vi "Day 19-1.vi"() -> ()   [LabVIEW 2020]
uses:
  Vec3.ctl
panel:
  out "Sensors - 1":i32
  out "Iterations":i32
  out "Max Manhattan Distance":dbl
  out "Beacon Count":i32
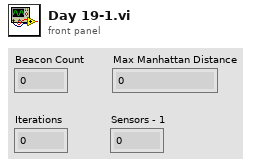
[diagram p1: front panel]
types:
  T1 = typedef "Vec3.ctl" = cluster{"X":dbl, "Y":dbl, "Z":dbl}
  T2 = typedef "Scanner.ctl" = cluster{"Position":T1, "Beacons":T1[]}
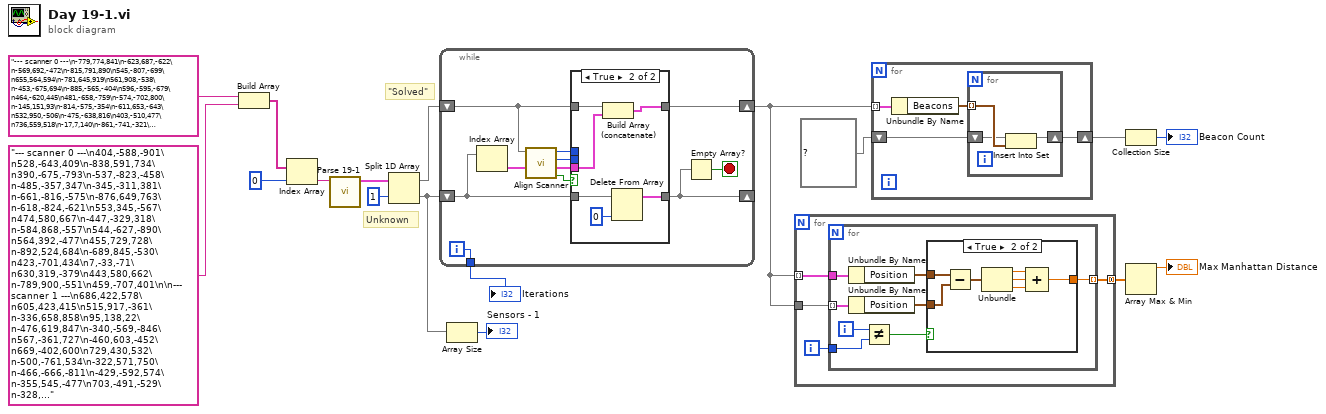
[diagram p0: block diagram]
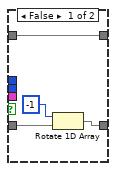
[diagram p3: hidden frame]
diagram:
  # "Unknown"
  # "\"Solved\""
  n1 = Build Array("--- scanner 0 ---\n-779,774,841\n-623,687,-622\n-569,692,-472\n-815,791,890\n545,-807,-699\n655,564,594\n-781,645,919\n561,908,-538\n-453,-675,694\n-885,-565,-404\n596,-595,-679\n464,-620,445\n481,-658,-759\n-574,-702,800\n-145,151,93\n-814,-575,-354\n-611,653,-643\n532,950,-506\n-475,-638,816\n403,-510,477\n736,559,518\n-17,7,140\n-861,-741,-321\n513,-554,586\n518,512,519\n549,924,-562\n\n--- scanner 1 ---\n689,772,-758\n537,371,685\n-672,-658,689\n123,51,-21\n-401,435,-501\n12,-98,95\n735,588,-720\n844,-573,-785\n-423,-889,-362\n-816,-649,595\n655,605,-727\n785,-703,-813\n536,-624,720\n-360,-902,-383\n-432,400,599\n-689,-669,583\n625,506,710\n455,445,698\n650,-556,751\n747,-531,-750\n-346,-875,-402\n-417,420,420\n-501,413,-386\n490,-584,661\n-499,374,505\n-449,476,-453\n\n--- scanner 2 ---\n663,667,-407\n-595,-818,-576\n-309,605,562\n-598,-610,-587\n-517,-586,691\n46,-151,22\n-881,281,-669\n732,-947,-380\n587,624,746\n-55,-3,100\n-458,-497,709\n593,687,-248\n572,498,738\n694,-939,-344\n401,-634,682\n-847,239,-653\n397,-527,600\n-610,-743,-467\n-474,659,598\n-414,-596,646\n657,542,-317\n-397,630,676\n378,-659,657\n-848,236,-666\n514,509,638\n753,-870,-512\n\n--- scanner 3 ---\n438,673,-607\n-400,-430,341\n-795,-514,-738\n-705,-416,-761\n760,-806,792\n-469,803,349\n670,-798,675\n363,648,-428\n-349,-447,506\n-425,412,-482\n520,455,660\n452,-616,-878\n553,372,771\n24,68,-59\n654,413,728\n-464,-413,481\n-404,598,-552\n-459,781,522\n538,-597,-851\n-346,488,-476\n420,-481,-842\n-470,896,540\n651,-822,721\n421,522,-506\n-690,-511,-769\n\n--- scanner 4 ---\n844,592,402\n-636,679,516\n-720,-400,911\n-509,-714,-788\n-826,755,-326\n39,-121,70\n661,741,-539\n727,636,527\n869,-741,-241\n742,-762,619\n-703,-565,962\n725,-852,686\n-639,710,621\n829,579,592\n654,730,-279\n-737,-540,847\n-734,702,606\n-487,-705,-778\n799,-689,-246\n-754,837,-380\n854,-715,-315\n754,-648,701\n-615,725,-335\n-628,-713,-672\n736,727,-443\n\n--- scanner 5 ---\n-405,590,-366\n-409,651,-375\n439,489,371\n-542,-507,536\n-367,404,-381\n299,-367,848\n-670,-452,-700\n-49,132,11\n340,-226,895\n478,-800,-337\n613,500,-723\n279,-348,939\n-558,-502,654\n390,411,415\n366,500,429\n400,-731,-350\n-612,-578,-728\n629,662,-720\n-522,-490,-688\n-453,406,393\n-679,460,405\n-652,411,356\n-532,-505,547\n707,591,-772\n635,-703,-379\n\n--- scanner 6 ---\n539,-841,504\n743,731,-445\n-822,-423,673\n-770,-492,627\n-762,805,536\n622,783,749\n-757,320,-629\n710,684,-611\n393,-892,456\n-769,705,691\n365,-675,-379\n-831,401,-736\n561,779,740\n-815,623,585\n385,-726,-591\n305,-611,-528\n-26,-6,-67\n-690,441,-682\n-830,-855,-756\n-707,-427,667\n808,821,734\n660,755,-621\n444,-961,435\n-831,-858,-732\n-873,-889,-537\n-116,-144,21\n\n--- scanner 7 ---\n620,-673,-810\n601,-454,-802\n-496,543,-614\n-596,554,-672\n963,-487,692\n-701,-396,401\n808,816,748\n638,-546,-875\n887,-534,765\n-604,428,-687\n916,-611,754\n-456,393,374\n-554,-588,-462\n549,385,-763\n-420,447,209\n-784,-504,377\n811,771,781\n-510,-687,-472\n-725,-524,511\n459,510,-757\n795,813,747\n71,-145,-43\n390,365,-693\n-534,422,297\n-565,-706,-544\n122,13,-148\n\n--- scanner 8 ---\n300,838,-511\n723,-429,-827\n-489,-531,-733\n-862,690,478\n272,779,-641\n365,729,650\n-749,-606,618\n-412,-399,-712\n-420,-363,-674\n-763,627,434\n584,-407,497\n-725,663,-381\n702,-366,-840\n358,649,667\n-832,581,-377\n683,-352,-813\n-773,672,537\n699,-507,475\n-616,-486,630\n-700,638,-358\n327,683,834\n632,-455,538\n335,741,-469\n-541,-595,615\n-76,130,123\n\n--- scanner 9 ---\n643,-906,-639\n554,-930,-576\n-438,-780,848\n885,648,-659\n-617,748,624\n708,-887,-479\n562,675,352\n513,-416,680\n-551,607,575\n867,701,-509\n567,599,433\n-593,592,-482\n533,-475,546\n-618,-692,-723\n-629,538,-371\n928,733,-581\n116,-32,-131\n405,-499,656\n515,674,570\n-629,-736,-551\n71,-144,33\n-384,-744,683\n-655,512,-481\n-658,-823,-634\n-413,-666,760\n-507,716,685\n\n--- scanner 10 ---\n392,400,680\n715,-577,488\n872,575,-780\n-527,-916,-745\n-756,759,-452\n-341,-954,-730\n360,461,570\n553,-799,-423\n-489,-888,625\n731,-478,552\n-844,478,532\n609,-456,515\n777,572,-702\n-439,-817,615\n641,-709,-383\n501,510,636\n-705,828,-431\n-764,593,595\n-610,708,-500\n-406,-864,449\n-77,-136,-15\n515,-651,-411\n-588,-912,-736\n1,17,72\n844,455,-646\n-784,542,383\n\n--- scanner 11 ---\n-705,-729,760\n-796,-680,666\n34,174,59\n681,672,720\n-634,-677,682\n685,-381,-430\n736,900,-429\n-892,-338,-314\n-28,77,-93\n-796,472,419\n731,-487,-512\n-885,399,-599\n746,727,-451\n-885,458,443\n678,-536,-330\n652,-373,448\n666,-453,483\n-706,-323,-352\n-807,414,492\n734,-275,479\n602,750,578\n-890,436,-400\n591,761,630\n-645,-332,-356\n-836,448,-626\n735,709,-336\n\n--- scanner 12 ---\n560,-631,663\n3,-21,-120\n425,-576,-600\n455,612,-831\n-472,492,-534\n615,888,330\n-382,383,326\n414,511,-837\n76,90,15\n-423,476,-725\n-568,-599,563\n751,919,441\n480,-626,-579\n-464,570,-714\n425,438,-790\n-744,-590,-577\n461,-722,-487\n-459,-674,578\n-688,-533,-461\n-366,425,292\n-369,380,325\n-448,-466,575\n597,-635,584\n647,-481,631\n753,946,365\n-709,-755,-482\n\n--- scanner 13 ---\n-793,-712,526\n43,-66,-77\n-592,814,658\n608,-557,-325\n-817,-758,545\n-447,441,-677\n-476,805,776\n377,-808,643\n685,332,-669\n-306,539,-675\n-533,-777,-578\n527,469,775\n576,-489,-523\n666,440,-717\n418,-765,542\n-678,-863,-623\n623,-570,-556\n-625,-783,-492\n460,-697,676\n653,391,833\n-611,841,744\n774,405,-693\n-801,-829,436\n678,570,758\n-11,91,43\n-418,455,-584\n\n--- scanner 14 ---\n805,-443,-751\n494,718,482\n2,-16,82\n104,91,-72\n-597,622,-615\n-753,481,430\n-531,502,409\n-672,731,-630\n-588,446,525\n571,-495,655\n-464,742,-627\n385,808,-378\n751,-407,-916\n382,821,-377\n-351,-554,-767\n-338,-407,491\n560,-451,483\n-450,-491,-811\n478,767,673\n531,-364,566\n-440,-536,-708\n-297,-435,349\n776,-521,-828\n572,726,662\n427,824,-344\n-266,-423,363\n\n--- scanner 15 ---\n-459,-573,-393\n-541,-681,657\n-691,578,-927\n846,-686,740\n854,-755,-493\n-670,527,-858\n-18,154,-79\n540,944,-704\n-392,942,855\n-622,673,-807\n-435,-635,739\n-453,-688,-389\n673,-696,718\n689,-806,-510\n549,934,-726\n345,935,570\n541,828,-585\n122,-41,-59\n-499,-636,-458\n382,940,769\n-377,756,817\n714,-691,-476\n-590,-628,839\n655,-685,833\n-386,695,813\n394,886,543\n\n--- scanner 16 ---\n729,789,-842\n-819,-334,502\n-741,-438,568\n399,-785,-551\n682,756,-676\n753,706,-666\n-9,-118,-9\n318,-711,-658\n-857,-784,-531\n439,-644,-605\n-891,-827,-750\n479,467,552\n659,-682,340\n-106,61,-102\n-681,548,823\n-664,604,849\n-860,-785,-555\n-613,351,-759\n-677,411,-908\n550,-780,387\n-728,431,-696\n-844,-469,484\n437,638,591\n-693,572,807\n491,488,586\n669,-789,409\n\n--- scanner 17 ---\n-418,-800,568\n690,-779,507\n441,-370,-505\n-573,-900,575\n-327,-603,-487\n552,-453,-472\n863,-801,517\n-436,328,515\n420,808,-712\n731,415,512\n-524,-718,522\n491,824,-603\n-18,24,64\n109,-51,-38\n-303,-536,-502\n-677,620,-677\n-482,397,567\n537,800,-622\n-442,332,630\n706,449,397\n484,-411,-606\n672,-894,518\n-576,655,-745\n871,432,448\n-517,524,-688\n-258,-444,-547\n\n--- scanner 18 ---\n-674,750,495\n-412,-547,817\n610,-432,859\n-410,-437,-273\n648,612,-461\n-691,786,446\n738,446,520\n-464,-684,742\n637,554,-561\n-494,402,-503\n33,115,-7\n775,424,642\n-612,484,-492\n541,-269,-637\n-545,752,417\n720,-493,891\n-430,-571,-332\n487,-434,-601\n-31,4,175\n802,545,536\n654,-542,750\n-302,-461,-356\n516,-357,-523\n522,627,-453\n-459,-765,818\n-593,412,-547\n\n--- scanner 19 ---\n-62,159,-61\n396,-693,-479\n-641,729,543\n-709,-486,661\n-552,-810,-705\n-796,708,-772\n-656,620,468\n522,-264,566\n-653,609,676\n-662,-436,507\n360,-565,-518\n-774,808,-657\n7,-11,2\n419,-516,-543\n409,-300,420\n352,889,-418\n383,849,609\n341,867,-488\n406,888,-551\n-733,760,-705\n501,-319,516\n-741,-399,511\n404,870,387\n499,905,552\n-725,-728,-734\n-597,-770,-717\n\n--- scanner 20 ---\n-649,836,908\n463,700,656\n552,809,589\n524,739,-436\n758,-723,501\n528,-639,-338\n484,-540,-348\n-914,776,-711\n-716,790,773\n-942,-616,878\n4,117,4\n-627,-773,-678\n-917,764,-831\n376,757,614\n-810,864,802\n699,-703,635\n-646,-554,-686\n539,-521,-420\n579,871,-390\n675,-831,525\n-184,-41,64\n-950,617,-725\n-664,-681,-751\n-989,-740,816\n-913,-693,889\n610,802,-431\n\n--- scanner 21 ---\n-328,515,-481\n-417,574,-499\n-621,584,416\n-465,-344,-508\n595,590,900\n793,-530,-444\n-358,-340,-590\n-386,-522,745\n154,-26,152\n-358,-580,619\n705,529,868\n50,99,-7\n799,454,-514\n540,-327,651\n577,-349,529\n-755,704,388\n-427,471,-544\n661,639,759\n774,366,-628\n-490,-321,-533\n513,-448,545\n-677,701,483\n-398,-670,707\n667,-515,-452\n678,-457,-552\n828,531,-592\n\n--- scanner 22 ---\n-354,917,781\n-281,841,734\n639,-856,-861\n562,853,614\n600,-872,-861\n650,-340,634\n-669,-830,764\n615,792,515\n-514,-535,-659\n-645,-747,872\n566,-839,-856\n-581,-624,-768\n399,493,-762\n-262,577,-795\n535,464,-683\n391,829,533\n-535,-771,744\n-368,738,-823\n-397,644,-749\n74,32,12\n587,-316,723\n490,-359,569\n-292,870,657\n549,579,-709\n-556,-448,-716\n\n--- scanner 23 ---\n-854,-686,494\n471,874,648\n488,-734,-887\n764,427,-727\n-759,681,-745\n-725,-714,449\n-605,728,-695\n795,538,-591\n458,-463,533\n405,770,623\n387,-740,-928\n-843,-741,525\n477,-316,412\n-885,549,507\n-750,-482,-862\n822,462,-589\n-158,-21,43\n461,812,673\n-755,760,-782\n-166,125,-115\n448,-380,515\n-700,-503,-917\n-884,648,444\n-824,602,404\n-846,-390,-881\n314,-693,-917\n\n--- scanner 24 ---\n-886,423,811\n785,453,423\n-396,553,-508\n-81,38,127\n-415,618,-348\n-522,-528,979\n706,-897,440\n-479,-748,-503\n652,-801,-610\n-610,-708,-592\n603,-785,-419\n611,-707,-599\n693,-894,441\n861,406,496\n736,672,-473\n-636,-503,891\n-372,464,-445\n814,530,434\n-29,-119,-2\n-558,-474,814\n-803,315,787\n773,654,-249\n-566,-719,-420\n709,-852,407\n797,573,-420\n-827,443,677\n\n--- scanner 25 ---\n-729,-745,477\n-809,409,-655\n628,-585,534\n405,464,-835\n309,581,335\n-697,-756,-375\n-459,599,568\n-390,539,409\n-626,-825,-487\n-823,-783,491\n340,-640,-575\n-14,-66,28\n-435,584,501\n334,-554,-667\n420,614,418\n352,480,376\n-157,-24,-97\n560,-387,566\n254,-685,-720\n359,483,-859\n-649,398,-559\n-616,-862,-402\n547,-618,581\n-708,341,-690\n288,374,-843\n-751,-815,603\n\n--- scanner 26 ---\n409,289,-495\n-847,-575,496\n413,467,-563\n508,-736,-627\n-930,-464,529\n530,380,608\n-764,280,526\n628,-869,503\n-42,-169,-23\n650,-658,-548\n503,274,552\n624,-954,561\n-499,-886,-493\n-406,-695,-494\n-856,235,571\n560,-747,-638\n-400,550,-551\n-889,-507,630\n-500,395,-544\n-521,-713,-483\n-582,501,-498\n-697,304,511\n440,253,530\n-170,-6,-82\n378,387,-577\n649,-801,614\n\n--- scanner 27 ---\n367,-847,-431\n805,450,827\n-651,-490,-341\n574,-485,737\n86,-58,110\n706,386,811\n-461,301,-317\n-745,-441,-432\n419,347,-310\n827,413,705\n-667,-493,-503\n329,-832,-245\n466,513,-343\n-529,329,473\n-599,353,-300\n-438,-863,890\n-541,433,385\n-516,-876,959\n371,-838,-492\n-673,-834,862\n632,-513,611\n-573,307,-497\n484,-525,649\n395,523,-393\n-513,468,378\n\n--- scanner 28 ---\n-568,386,784\n20,-72,121\n-121,24,13\n544,777,598\n-450,-510,942\n778,-914,-767\n830,-551,427\n-470,476,807\n-501,832,-460\n-378,-456,860\n358,756,528\n-717,-908,-600\n552,-860,-755\n790,-530,473\n-589,-465,830\n579,-909,-804\n-484,781,-295\n750,-556,440\n434,835,522\n-576,-802,-608\n727,722,-476\n-565,491,815\n-467,717,-435\n749,712,-303\n842,711,-494\n-695,-918,-609\n\n--- scanner 29 ---\n417,-415,713\n-449,647,870\n27,91,28\n402,-451,-539\n476,382,916\n-393,704,754\n548,-455,624\n-428,869,849\n857,539,-539\n-777,-601,-329\n-126,-2,126\n-665,-378,797\n827,434,-697\n-541,876,-635\n319,-462,-354\n504,-444,796\n-462,887,-670\n-714,-362,606\n-673,-456,617\n460,454,788\n488,413,930\n-888,-669,-268\n842,448,-606\n-852,-520,-276\n400,-532,-343\n-583,781,-617\n\n--- scanner 30 ---\n397,-399,-587\n-692,640,606\n-549,-426,-591\n517,-468,-682\n503,792,687\n-665,724,474\n683,415,-508\n469,573,730\n-665,-505,-567\n-470,730,-541\n632,627,-528\n747,564,-448\n466,-420,-536\n72,63,-118\n935,-637,679\n-375,-466,480\n-385,-494,361\n931,-631,564\n866,-591,627\n500,768,688\n-305,727,-516\n-647,841,608\n-776,-459,-594\n-413,713,-575\n-379,-503,254\n\n--- scanner 31 ---\n-626,-772,665\n-298,775,-361\n795,558,497\n-650,-716,745\n470,819,-606\n-465,-720,-367\n783,706,535\n476,861,-359\n426,-668,854\n16,67,24\n-559,670,547\n59,-95,-131\n754,-852,-774\n775,-921,-723\n560,-548,826\n-456,-698,-357\n823,616,623\n-452,696,550\n706,-801,-628\n-457,-579,-473\n-310,549,-415\n-441,686,552\n504,-665,759\n461,823,-545\n-755,-747,659\n-261,576,-366\n\n--- scanner 32 ---\n908,721,721\n86,-57,-97\n-713,-299,-592\n-758,-783,430\n-779,-597,500\n818,456,-829\n-623,521,428\n-837,-707,424\n907,-562,-902\n549,-311,329\n528,-351,375\n860,594,720\n-655,405,401\n-714,-392,-401\n829,529,-887\n912,-363,-865\n554,-391,342\n695,675,687\n-724,-414,-574\n-659,757,-629\n-69,-11,3\n-569,667,-540\n-586,448,388\n-580,615,-551\n907,480,-843\n858,-589,-853\n\n--- scanner 33 ---\n-779,-614,345\n695,317,397\n-753,576,801\n505,341,-394\n411,432,-345\n-667,-708,-706\n615,-385,529\n643,-378,564\n557,300,449\n-879,-666,355\n483,-862,-738\n-112,-148,91\n489,503,-397\n718,-890,-767\n-711,-622,-690\n-721,-601,-807\n-870,-758,402\n33,-26,-17\n-604,557,-459\n640,-959,-780\n-592,444,-618\n627,-473,425\n-758,670,920\n-605,562,-647\n583,497,403\n-870,560,878", "--- scanner 0 ---\n404,-588,-901\n528,-643,409\n-838,591,734\n390,-675,-793\n-537,-823,-458\n-485,-357,347\n-345,-311,381\n-661,-816,-575\n-876,649,763\n-618,-824,-621\n553,345,-567\n474,580,667\n-447,-329,318\n-584,868,-557\n544,-627,-890\n564,392,-477\n455,729,728\n-892,524,684\n-689,845,-530\n423,-701,434\n7,-33,-71\n630,319,-379\n443,580,662\n-789,900,-551\n459,-707,401\n\n--- scanner 1 ---\n686,422,578\n605,423,415\n515,917,-361\n-336,658,858\n95,138,22\n-476,619,847\n-340,-569,-846\n567,-361,727\n-460,603,-452\n669,-402,600\n729,430,532\n-500,-761,534\n-322,571,750\n-466,-666,-811\n-429,-592,574\n-355,545,-477\n703,-491,-529\n-328,-685,520\n413,935,-424\n-391,539,-444\n586,-435,557\n-364,-763,-893\n807,-499,-711\n755,-354,-619\n553,889,-390\n\n--- scanner 2 ---\n649,640,665\n682,-795,504\n-784,533,-524\n-644,584,-595\n-588,-843,648\n-30,6,44\n-674,560,763\n500,723,-460\n609,671,-379\n-555,-800,653\n-675,-892,-343\n697,-426,-610\n578,704,681\n493,664,-388\n-671,-858,530\n-667,343,800\n571,-461,-707\n-138,-166,112\n-889,563,-600\n646,-828,498\n640,759,510\n-630,509,768\n-681,-892,-333\n673,-379,-804\n-742,-814,-386\n577,-820,562\n\n--- scanner 3 ---\n-589,542,597\n605,-692,669\n-500,565,-823\n-660,373,557\n-458,-679,-417\n-488,449,543\n-626,468,-788\n338,-750,-386\n528,-832,-391\n562,-778,733\n-938,-730,414\n543,643,-506\n-524,371,-870\n407,773,750\n-104,29,83\n378,-903,-323\n-778,-728,485\n426,699,580\n-438,-605,-362\n-469,-447,-387\n509,732,623\n647,635,-688\n-868,-804,481\n614,-800,639\n595,780,-596\n\n--- scanner 4 ---\n727,592,562\n-293,-554,779\n441,611,-461\n-714,465,-776\n-743,427,-804\n-660,-479,-426\n832,-632,460\n927,-485,-438\n408,393,-506\n466,436,-512\n110,16,151\n-258,-428,682\n-393,719,612\n-211,-452,876\n808,-476,-593\n-575,615,604\n-485,667,467\n-680,325,-822\n-627,-443,-432\n872,-547,-609\n833,512,582\n807,604,487\n839,-516,451\n891,-625,532\n-652,-548,-490\n30,-46,-14") -> (w15:string[])
  n2 = Index Array(array=w15, index=0) -> (element=w13:string)
  n3 = call "Parse 19-1.vi"("String"=w13) -> ("Scanners"=w12:T2[])  [unwired: 10 in]
  n4 = Split 1D Array(array=w12, index=1) -> (first subarray=w10:T2[], second subarray=w2:T2[])
  n5 = while {
    shift-right: [w24] -> w6
    shift-left: w10 -> [w25]
    shift-right: [w23] -> _
    shift-left: w2 -> [w27]
    tunnel: [w18] -> w3
    i -> [w18]
    stop <- w22 stop-if-true
    n6 = Index Array(array=w27) -> (element=w28:T2)  [unwired: 1 in]
    n7 = call "Align Scanner.vi"("New Scanner"=w28, "Known Scanners"=w25) -> ("Aligned?"=w21:bool, "Updated Scanner"=w26:T2, "Best Scanner Index"=w19:i32, "Max Overlap"=w20:i32)  [unwired: 6 in]
    n8 = case shown="True" w21 {
      tunnel: w27 -> [w31 w35]
      tunnel: w26 -> [_ w37]
      tunnel: w25 -> [w32 w38]
      tunnel: [w32 w36] -> w24
      tunnel: [w29 w33] -> w23
      tunnel: w20 -> [_ _]
      tunnel: w19 -> [_ _]
      frame False {
        n9 = Rotate 1D Array(1:w31, 2:-1 ("n")) -> (0:w29:T2[])
      }
      frame True {
        n10 = Build Array (concatenate)(w38, w37) -> (w36:T2[])
        n11 = Delete From Array(array=w35, index=0) -> (array with subset deleted=w33:T2[])  [unwired: 1 in, 1 out]
      }
    }
    n12 = Empty Array?(array=w23) -> (empty?=w22:bool)
  }
  "Iterations" <- w3
  n13 = Array Size(array=w2) -> (size(s)=→"Sensors - 1":i32)
  n14 = for {
    tunnel: w6 -> [w42] mode=indexing
    tunnel: w6 -> [w41]
    tunnel: [w39] -> w5 mode=concatenating
    i -> [w40]
    n15 = for {
      tunnel: w42 -> [w50]
      tunnel: w41 -> [w49] mode=indexing
      tunnel: w40 -> [w47]
      tunnel: [w43] -> w39 mode=indexing
      i -> [w48]
      n16 = Unbundle By Name(w50) -> ("Position"=w44:T1)
      n17 = Unbundle By Name(w49) -> ("Position"=w45:T1)
      n18 = Not Equal?(x=w48, y=w47) -> (x != y?=w46:bool)
      n19 = case shown="True" w46 {
        tunnel: w45 -> [_ w56]
        tunnel: w44 -> [_ w57]
        tunnel: [_ w51] -> w43
        frame False {
        }
        frame True {
          n20 = Subtract(x=w57, y=w56) -> (x-y=w55:T1)
          n21 = Unbundle(w55) -> ("X"=w54:dbl, "Y"=w53:dbl, "Z"=w52:dbl)
          n22 = Compound Arithmetic op=ADD(w54, w53, w52) -> (w51:dbl)
        }
      }
    }
  }
  n23 = for {
    tunnel: w6 -> [w61] mode=indexing
    shift-right: [w58] -> w8
    shift-left: set{T1} {} ("set out") -> [w59]
    n24 = Unbundle By Name(w61) -> ("Beacons"=w60:T1[])
    n25 = for {
      tunnel: w60 -> [w64] mode=indexing
      shift-right: [w62] -> w58
      shift-left: w59 -> [w63]
      n26 = Insert Into Set(10:w64, 11:w63) -> (3:w62:set{T1})  [unwired: 1 out]
    }
  }
  n27 = Collection Size(1:w8) -> (0:→"Beacon Count":i32)
  n28 = Array Max & Min(array=w5) -> (max value=→"Max Manhattan Distance":dbl)  [unwired: 3 out]
